vi "Initialize.vi"(8 "error in (no error)":errorcluster, 11 "file handler in":refnum<class "File Handler.lvclass">) -> (0 "error out":errorcluster, 3 "file handler out":refnum<class "File Handler.lvclass">)   [LabVIEW 2024, in "Logging.lvlib" / "File Handler.lvclass"]
uses:
  File Handler.lvclass
  File Handler.lvclass/File Handler.ctl
  <vilib>/MakerHub/Toolbox/LMH-Toolbox.lvlib
panel:
  # "Connector Pane"
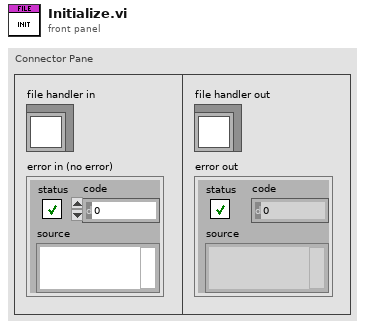
[diagram p1: front panel]
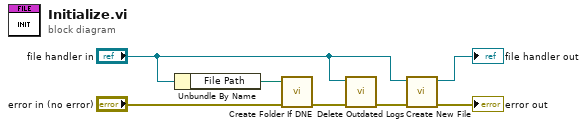
[diagram p0: block diagram]
diagram:
  n1 = Unbundle By Name("file handler in") -> ("File Path"=w4:path)
  n2 = call <vilib>:"Create Folder If DNE.vi"("Error In"="error in (no error)", "Folder Path"=w4) -> ("Error Out"=w3:errorcluster)  [unwired: 8 in, 1 out]
  n3 = call "Delete Outdated Logs.vi"("error in (no error)"=w3, "file handler in"="file handler in") -> ("error out"=w2:errorcluster)  [unwired: 9 in]
  n4 = call "Create New File.vi"("error in (no error)"=w2, "file handler in"="file handler in") -> ("error out"=→"error out":errorcluster, "file handler out"=→"file handler out":refnum<class "File Handler.lvclass">)  [unwired: 8 in]
